vi "Write JSON Config.vi"(6 "Pretty Print?":bool, 8 "error in (no error)":errorcluster, 11 "StringLen_I32 in":refnum<class "StringLen_I32.lvclass">) -> (0 "error out":errorcluster, 2 "JSON":string, 3 "StringLen_I32 out":refnum<class "StringLen_I32.lvclass">)   [LabVIEW 2021, in "StringLen_I32.lvclass"]
uses:
  StringLen_I32.lvclass
  C:/Program Files (x86)/National Instruments/LabVIEW 2021/vi.lib/TSA/Abstract Data Classes/Abs_Types/Type/Abs_Type.lvclass
  StringLen_I32.lvclass/StringLen_I32.ctl
  <vilib>/JDP Science/JSONtext/Make JSON Array.vi
  <vilib>/JDP Science/JSONtext/Merge into Object.vi
  <vilib>/JDP Science/JSONtext/Make JSON Object.vi
  <vilib>/Utility/LVClass/Get LV Class Name.vi
  <vilib>/JDP Science/JSONtext/support/Format JSON Array Text.vi
  <vilib>/JDP Science/JSONtext/support/Format JSON Object.vi
  <vilib>/JDP Science/JSONtext/Get all Object Items.vi
  <vilib>/JDP Science/JSONtext/Set Multiple Object Items.vi
  Abs_Types/String/Abs_String.lvclass
  Abs_Types/I32 Integer/Abs_I32 Integer.lvclass
  Abs_Types/Type/Abs_Type.lvclass
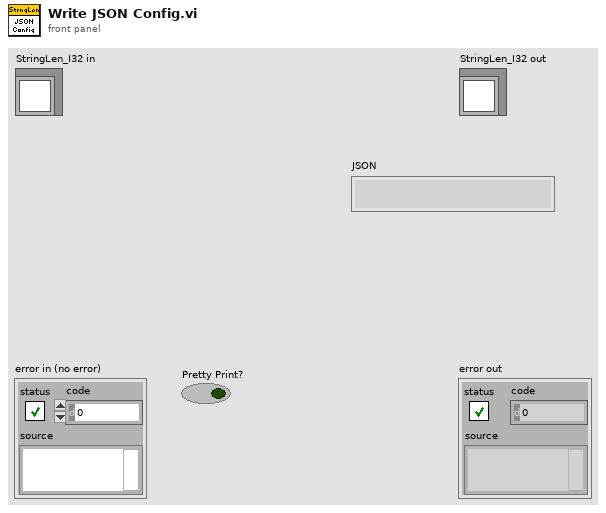
[diagram p1: front panel]
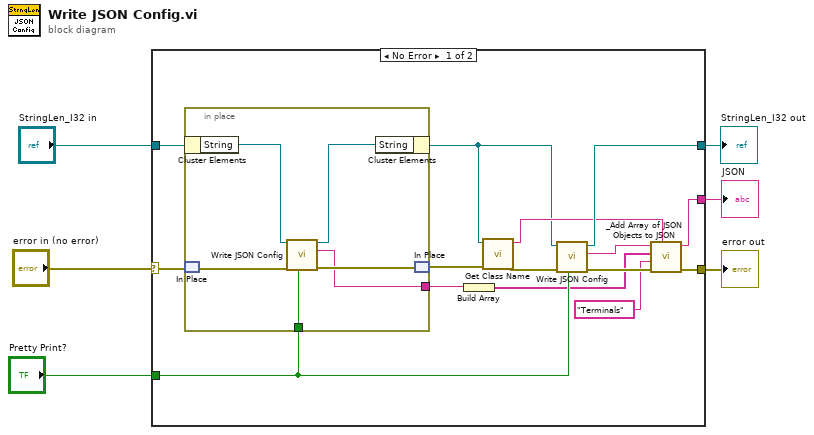
[diagram p0: block diagram]
diagram:
  n1 = case shown="No Error" "error in (no error)" {
    selector: "error in (no error)" -> [w11 w28]
    tunnel: [w21 w29] -> w6
    tunnel: [w19 w28] -> w5
    tunnel: [w17 _] -> w4
    tunnel: "StringLen_I32 in" -> [w13 w29]
    tunnel: "Pretty Print?" -> [w10 _]
    frame No Error {
      n2 = in-place {
        in-place-border: w10 -> [w26]
        in-place-border: [w24] -> w9
        n3 = in-place-cluster #1(w13) -> ("String"=w23:refnum<class "Abs_String.lvclass">)
        n4 = in-place-match #2(w11) -> (w27:errorcluster)
        n5 = call-dynamic "Write JSON Config.vi"("Pretty Print?"=w26, "error in (no error)"=w27, "Abs_Type in"=w23) -> ("error out"=w25:errorcluster, "JSON"=w24:string, "Abs_Type out"=w22:refnum<class "Abs_String.lvclass">)  [unwired: 6 in]
        n6 = in-place-cluster #1("String"=w22) -> (w12:refnum<class "StringLen_I32.lvclass">)
        n7 = in-place-match #2(w25) -> (w14:errorcluster)
      }
      n8 = Build Array(w9) -> (w8:string[])
      n9 = call "Get Class Name.vi"("error in (no error)"=w14, "Abs_Type in"=w12) -> ("error out"=w16:errorcluster, "class name"=w15:string)  [unwired: 8 in]
      n10 = call-parent "Write JSON Config.vi"("Pretty Print?"=w10, "error in (no error)"=w16, "Abs_Type in"=w12) -> ("error out"=w20:errorcluster, "JSON"=w18:string, "Abs_Type out"=w21:refnum<class "StringLen_I32.lvclass">)  [unwired: 6 in]
      n11 = call "_Add Array of JSON Objects to JSON.vi"("JSON Object Name"=w15, "error in (no error)"=w20, "JSON Array Name"="Terminals", "JSON Objects"=w8, "JSON"=w18) -> ("error out"=w19:errorcluster, "<JSON>"=w17:string)  [unwired: 5 in]
    }
    frame Error {
    }
  }
  "error out" <- w5
  "StringLen_I32 out" <- w6
  "JSON" <- w4
